vi "Calibration-Frame3.vi"(6 "Sampling speeds":T3={"Samples/ch"=600, "Sample Rate/ch (Hz)"=100.0} {"Sample Rate/ch (Hz)" min=0; "Samples/ch" min=0 step=1}, 7 "data mode":enum16{"Take new data point", "Refit Curve"}(ring), 9 "Fixed n":bool, 10 "Mode in":T2, 11 "Boolean in":bool) -> (1 "Sampling speeds Output":T1, 2 "Fixed n out":bool, 3 "Boolean out":bool)   [LabVIEW 2016]
uses:
  Anemometry Sub Vis/Calibration/Calib_mode.ctl
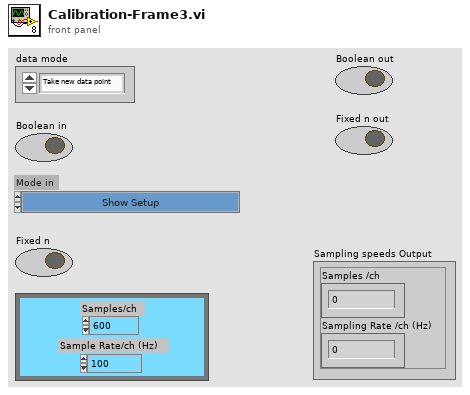
[diagram p1: front panel]
types:
  T1 = cluster{"Samples /ch":i32, "Sampling Rate /ch (Hz)":sgl}
  T2 = typedef "Calib_mode.ctl" = enum16{"Show Setup", "Take a New Calibration Point", "Refit Curve", "Setup Front Panel"}
  T3 = cluster{"Samples/ch":i32, "Sample Rate/ch (Hz)":sgl}
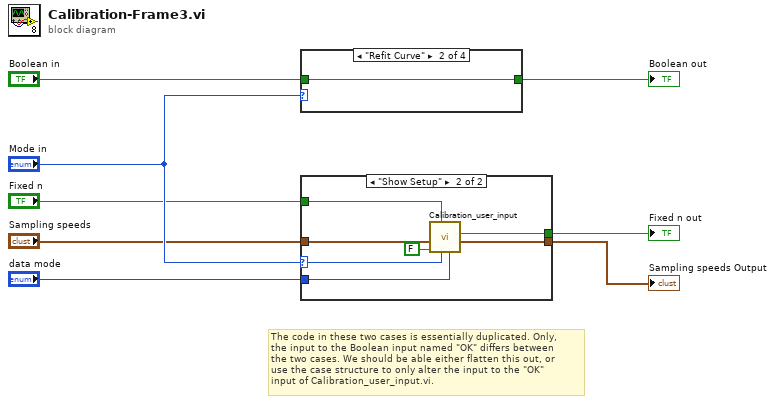
[diagram p0: block diagram]
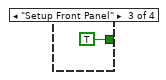
[diagram p3: hidden frame]
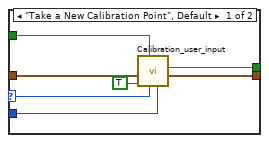
[diagram p5: hidden frame]
diagram:
  # "The code in these two cases is essentially duplicated. Only,\nthe input to the Boolean input named \"OK\" differs between\nthe two cases. We should be able either flatten this out, or\nuse the case structure to only alter the input to the \"OK\"\ninput of Calibration_user_input.vi."
  n1 = case shown="\"Refit Curve\"" "Mode in" {
    tunnel: [w9 w10 TRUE w12] -> w7
    tunnel: "Boolean in" -> [w9 w10 _ w12]
    frame "Show Setup" {
    }
    frame "Refit Curve" {
    }
    frame "Setup Front Panel" {
    }
    frame "Take a New Calibration Point" {
    }
  }
  "Boolean out" <- w7
  n2 = case shown="\"Show Setup\"" "Mode in" {
    selector: "Mode in" -> [w13 w20]
    tunnel: "Sampling speeds" -> [w19 w26]
    tunnel: "data mode" -> [w17 w24]
    tunnel: [w16 w23] -> w2
    tunnel: "Fixed n" -> [w14 w22]
    tunnel: [w15 w21] -> w4
    frame "Take a New Calibration Point", Default {
      n3 = call "Calibration_user_input.vi"("data mode"=w17, "Mode"=w13, "Fixed n"=w14, "OK"=TRUE, "Sampling speeds"=w19) -> ("Sampling speeds Output"=w16:T1, "Fixed n out"=w15:bool)  [unwired: 2 in, 3 out]
    }
    frame "Show Setup" {
      n4 = call "Calibration_user_input.vi"("data mode"=w24, "Mode"=w20, "Fixed n"=w22, "OK"=FALSE, "Sampling speeds"=w26) -> ("Sampling speeds Output"=w23:T1, "Fixed n out"=w21:bool)  [unwired: 5 out]
    }
  }
  "Fixed n out" <- w4
  "Sampling speeds Output" <- w2
